vi "Tosca-Process Event Accumulation.vi"(0 "accum state in":T2, 5 "state change":bool, 7 "Value in":bool, 9 "Accumulator":T1) -> (4 "accum state out":T2, 8 "Value out":bool)   [LabVIEW 2020]
uses:
  Typedefs/Tosca-Accumulator State.ctl
  Typedefs/Tosca-Accumulator.ctl
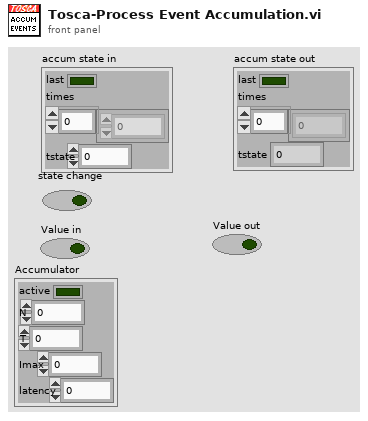
[diagram p1: front panel]
types:
  T1 = typedef "Tosca-Accumulator.ctl" = cluster{"active":bool, "N":i32, "T":dbl, "Imax":dbl, "latency":dbl}
  T2 = typedef "Tosca-Accumulator State.ctl" = cluster{"last":bool, "times":dbl[], "tstate":dbl}
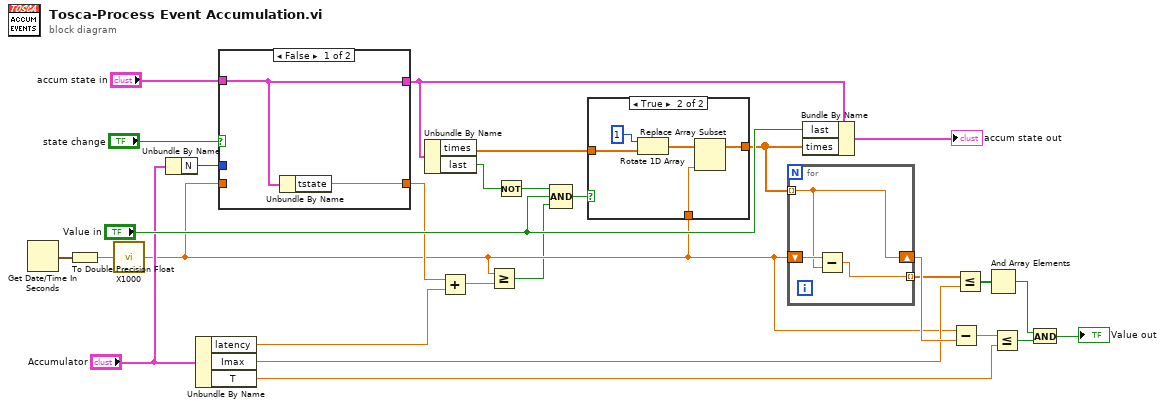
[diagram p0: block diagram]
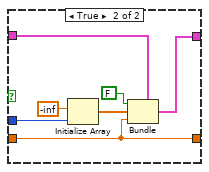
[diagram p2: hidden frame]
diagram:
  n1 = Get Date/Time In Seconds() -> (seconds since 1Jan1904=w22:timestamp)
  n2 = To Double Precision Float(number=w22) -> (double precision float=w19:dbl)
  n3 = call "X1000.vi"("X"=w19) -> ("X/1000"=w3:dbl)
  n4 = Unbundle By Name("Accumulator") -> ("N"=w7:i32)
  n5 = Unbundle By Name("Accumulator") -> ("latency"=w5:dbl, "Imax"=w13:dbl, "T"=w17:dbl)
  n6 = case shown="False" "state change" {
    tunnel: "accum state in" -> [w30 w32]
    tunnel: [w30 w33] -> w1
    tunnel: w7 -> [_ w34]
    tunnel: w3 -> [_ w31]
    tunnel: [w29 w31] -> w6
    frame False {
      n7 = Unbundle By Name(w30) -> ("tstate"=w29:dbl)
    }
    frame True {
      n8 = Initialize Array(-inf, w34) -> (w37:dbl[])
      n9 = Bundle(cluster=w32, "last"=FALSE, "times"=w37, "tstate"=w31) -> (w33:T2)
    }
  }
  n10 = Unbundle By Name(w1) -> ("times"=w26:dbl[], "last"=w28:bool)
  n11 = Add(x=w6, y=w5) -> (x+y=w4:dbl)
  n12 = Greater Or Equal?(x=w3, y=w4) -> (x >= y?=w2:bool)
  n13 = Not(x=w28) -> (.not. x?=w27:bool)
  n14 = Compound Arithmetic op=AND(w27, "Value in", w2) -> (w25:bool)
  n15 = case shown="True" w25 {
    tunnel: w26 -> [w38 w43]
    tunnel: [w38 w40] -> w21
    tunnel: w3 -> [_ w39]
    frame False {
    }
    frame True {
      n16 = Rotate 1D Array(1:w43, 2:1 ("n")) -> (0:w41:dbl[])
      n17 = Replace Array Subset(array=w41, new element=w39) -> (w40:dbl[])  [unwired: 1 in]
    }
  }
  n18 = for {
    tunnel: w21 -> [w45] mode=indexing
    shift-right: [w45] -> w20
    shift-left: w3 -> [w46]
    tunnel: [w44] -> w14 mode=indexing
    n19 = Subtract(x=w46, y=w45) -> (x-y=w44:dbl)
  }
  n20 = Bundle By Name(cluster=w1, "last"="Value in", "times"=w21) -> (→"accum state out":T2)
  n21 = Subtract(x=w3, y=w20) -> (x-y=w18:dbl)
  n22 = Less Or Equal?(x=w14, y=w13) -> (x <= y?=w12:bool[])
  n23 = And Array Elements(Boolean array=w12) -> (logical AND=w11:bool)
  n24 = Less Or Equal?(x=w18, y=w17) -> (x <= y?=w16:bool)
  n25 = And(x=w11, y=w16) -> (x .and. y?=→"Value out":bool)
